vi "Counter.vi"(0 "Counter End  Value":u32, 1 "Input Valid":bool=TRUE, 7 "Reset":bool) -> (4 "Counter Value":u32, 8 "End Reached":bool)   [LabVIEW 2014, in "DHT11 (FPGA).lvlib"]
uses:
  DHT11 (FPGA).lvlib
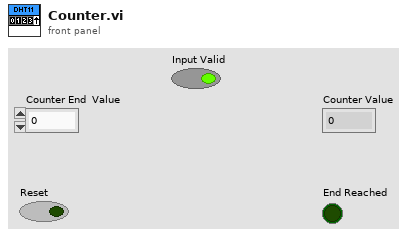
[diagram p1: front panel]
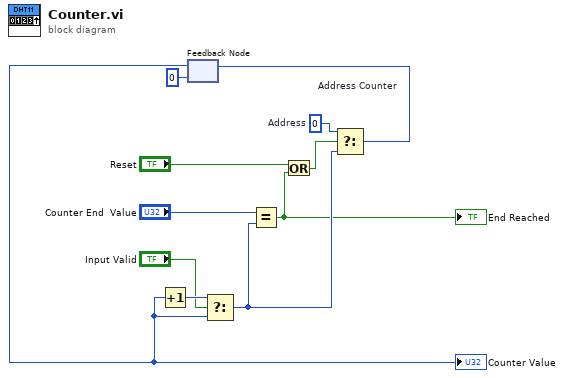
[diagram p0: block diagram]
diagram:
  w11 = u32 0  # Address
  n1 = feedback #1 "Address Counter"(u32 0 ("Address")) -> (w4:u32)
  "Counter Value" <- w4
  n2 = Increment(x=w4) -> (x+1=w8:u32)
  n3 = Select(t=w8, s="Input Valid", f=w4) -> (s? t:f=w7:u32)
  n4 = Equal?(x="Counter End  Value", y=w7) -> (x = y?=w2:bool)
  "End Reached" <- w2
  n5 = Or(x="Reset", y=w2) -> (x .or. y?=w3:bool)
  n6 = Select(t=w11, s=w3, f=w7) -> (s? t:f=w10:u32)
  n7 = feedback-in #1(w10) -> ()
